vi "Write Data.vi"(8 "error in (no error)":errorcluster, 9 "Publication Time":timestamp, 10 "Value":variant, 11 "TerminalEnabledStateBinding In":refnum<class "TerminalEnabledStateBinding.lvclass">) -> (0 "error out":errorcluster, 3 "TerminalEnabledStateBinding Out":refnum<class "TerminalEnabledStateBinding.lvclass">)   [LabVIEW 2018, in "MVA Framework.lvlib" / "TerminalEnabledStateBinding.lvclass"]
doc: "写入数据"
uses:
  TerminalEnabledStateBinding.lvclass
  TerminalPropertyBinding/TerminalPropertyBinding.lvclass
  <vilib>/ErrorRing/Error Ring.xnode
  <vilib>/Utility/error.llb/Error Cluster From Error Code.vi
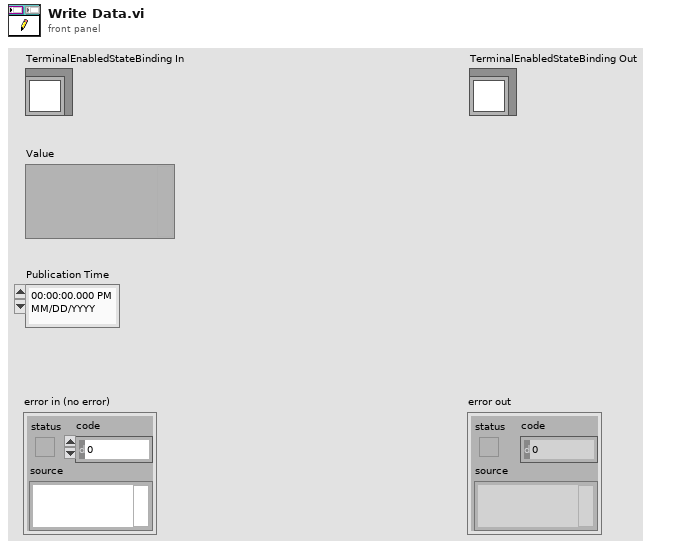
[diagram p1: front panel]
types:
  T1 = enum8{"Enabled", "Disabled", "Disabled and Grayed Out"}
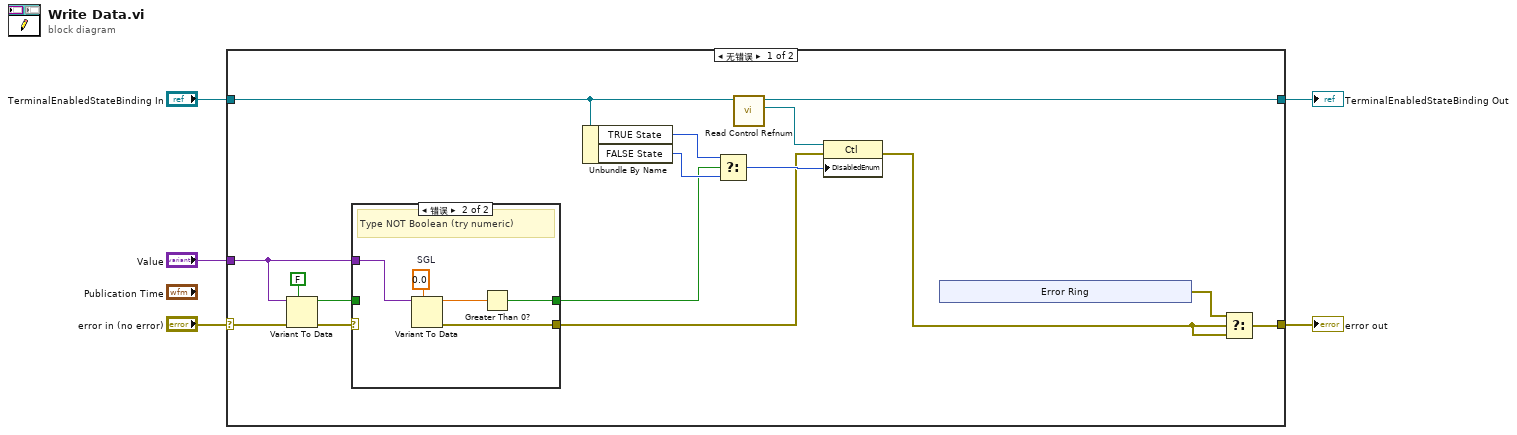
[diagram p0: block diagram]
diagram:
  n1 = case shown="无错误" "error in (no error)" {
    selector: "error in (no error)" -> [w14 w35]
    tunnel: "TerminalEnabledStateBinding In" -> [w9 w34]
    tunnel: "Value" -> [w17 _]
    tunnel: [w16 w34] -> w4
    tunnel: [w10 w35] -> w2
    frame No Error {
      n2 = Variant To Data(error in=w14, type=FALSE, Variant=w17) -> (data=w19:bool, error out=w18:errorcluster)
      n3 = case shown="错误" w18 {
        selector: w18 -> [w27 _]
        tunnel: w19 -> [w28 _]
        tunnel: [w28 w31] -> w6
        tunnel: w17 -> [_ w30]
        tunnel: [w27 w29] -> w13
        frame No Error {
          # "Type = Boolean (OK)"
        }
        frame Error {
          w33 = sgl 0.0  # SGL
          # "Type NOT Boolean (try numeric)"
          n4 = Variant To Data(type=w33, Variant=w30) -> (data=w32:sgl, error out=w29:errorcluster)  [unwired: 1 in]
          n5 = Greater Than 0?(x=w32) -> (x > 0?=w31:bool)
        }
      }
      n6 = Unbundle By Name(w9) -> ("TRUE State"=w8:T1, "FALSE State"=w7:T1)
      n7 = Select(t=w8, s=w6, f=w7) -> (s? t:f=w20:T1)
      n8 = call "Read Control Refnum.vi"("TerminalReferenceBinding in"=w9) -> ("Ctl Refnum"=w15:refnum<vi>, "TerminalReferenceBinding out"=w16:refnum<class "TerminalEnabledStateBinding.lvclass">)  [unwired: 9 in]
      n9 = property class="Ctl"(reference=w15, error in=w13, "DisabledEnum"=w20) -> (error out=w11:errorcluster)  [unwired: 1 out]
      n10 = xnode "Error Ring"() -> ("错误输出"=w12:errorcluster)
      n11 = Select(t=w12, s=w11, f=w11) -> (s? t:f=w10:errorcluster)
    }
    frame Error {
    }
  }
  "error out" <- w2
  "TerminalEnabledStateBinding Out" <- w4
